vi "rad_Create AppImage Info File.vi"(8 "error in (no error)":errorcluster, 10 "Temp Image Folder":path, 11 "AppImage Properties":T1) -> (0 "error out":errorcluster, 3 "App Image Info file path":path)   [LabVIEW 2020]
uses:
  TypeDefs/rad_Application Image Properties.ctl
  TypeDefs/rad_FPGA Properties.ctl
  TypeDefs/rad_FPGA Flash Properties.ctl
  rad_Globals.vi
  <vilib>/Utility/config.llb/Write Key (String).vi
  <vilib>/Utility/config.llb/NI_LVConfig.lvlib
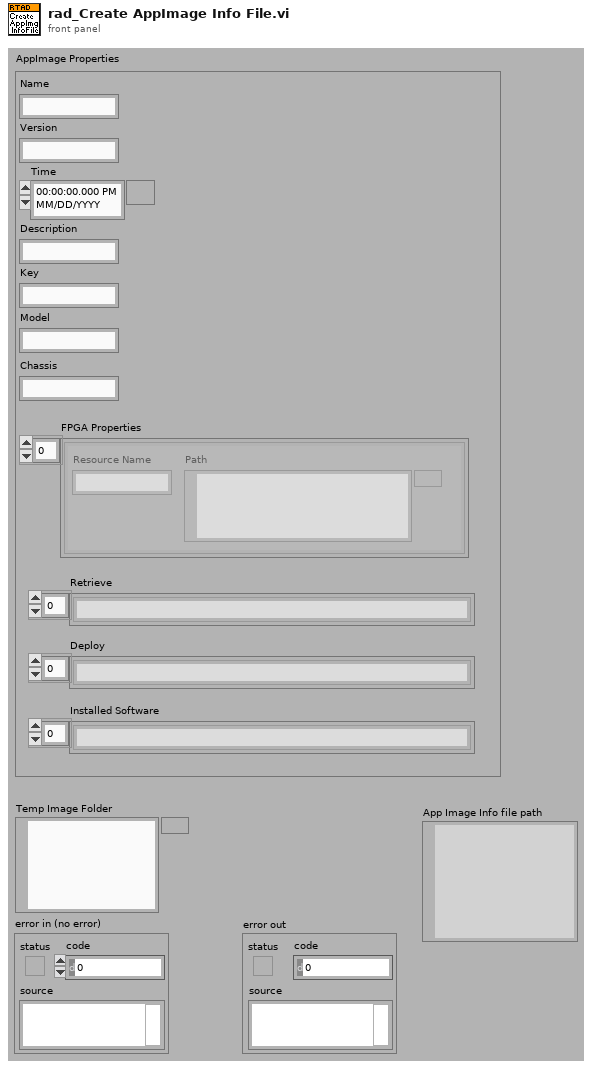
[diagram p1: front panel]
types:
  T1 = typedef "rad_Application Image Properties.ctl" = cluster{"Name":string, "Version":string, "Time":timestamp, "Description":string, "Key":string, "Chassis":string, "FPGA Properties":T2, "Model":string, "Retrieve":string[], "Deploy":string[], "Installed Software":string[]}
  T2 = typedef "rad_FPGA Properties.ctl" = T3[]
  T3 = typedef "rad_FPGA Flash Properties.ctl" = cluster{"Resource Name":string, "Path":path}
  T4 = typedef "NI_LVConfig.lvlib/Config Data RefNum.ctl" = refnum<k1>
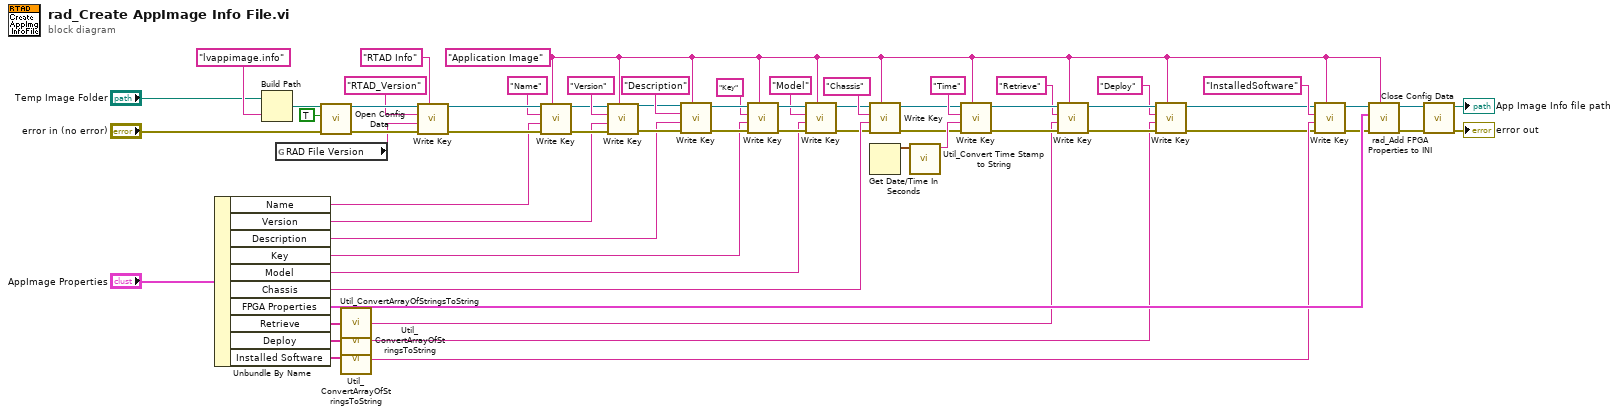
[diagram p0: block diagram]
diagram:
  w6 = "Application Image" ("section")
  n1 = Unbundle By Name("AppImage Properties") -> ("Name"=w41:string, "Version"=w40:string, "Description"=w30:string, "Key"=w29:string, "Model"=w21:string, "Chassis"=w31:string, "FPGA Properties"=w26:T2, "Retrieve"=w13:string[], "Deploy"=w12:string[], "Installed Software"=w8:string[])
  n2 = Build Path(base path="Temp Image Folder", name or relative path="lvappimage.info") -> (appended path=w53:path)
  n3 = global read "rad_Globals.vi" "RAD File Version"() -> (w38:string)
  n4 = call <vilib>:"Open Config Data.vi"("error in (no error)"="error in (no error)", "create file if necessary (T)"=TRUE, "configuration file path"=w53) -> ("error out"=w58:errorcluster, "refnum"=w57:T4)  [unwired: 6 in, 1 out]
  n5 = call "Util_ConvertArrayOfStringsToString.vi"("Array<string>"=w13) -> ("String"=w11:string)
  n6 = call "Util_ConvertArrayOfStringsToString.vi"("Array<string>"=w12) -> ("String"=w10:string)
  n7 = call "Util_ConvertArrayOfStringsToString.vi"("Array<string>"=w8) -> ("String"=w7:string)
  n8 = call-poly <vilib>:"Write Key.vi"("section"="RTAD Info", "error in (no error)"=w58, "value"=w38, "key"="RTAD_Version", "refnum"=w57) -> ("error out"=w59:errorcluster, "refnum out"=w60:T4)  [unwired: 1 in, 4 out]
  n9 = call-poly <vilib>:"Write Key.vi"("section"=w6, "error in (no error)"=w59, "value"=w41, "key"="Name", "refnum"=w60) -> ("error out"=w46:errorcluster, "refnum out"=w47:T4)  [unwired: 1 in, 4 out]
  n10 = call-poly <vilib>:"Write Key.vi"("section"=w6, "error in (no error)"=w46, "value"=w40, "key"="Version", "refnum"=w47) -> ("error out"=w49:errorcluster, "refnum out"=w50:T4)  [unwired: 1 in, 4 out]
  n11 = call-poly <vilib>:"Write Key.vi"("section"=w6, "error in (no error)"=w49, "value"=w30, "key"="Description", "refnum"=w50) -> ("error out"=w36:errorcluster, "refnum out"=w37:T4)  [unwired: 1 in, 4 out]
  n12 = call-poly <vilib>:"Write Key.vi"("section"=w6, "error in (no error)"=w36, "value"=w29, "key"="Key", "refnum"=w37) -> ("error out"=w23:errorcluster, "refnum out"=w25:T4)  [unwired: 1 in, 4 out]
  n13 = call-poly <vilib>:"Write Key.vi"("section"=w6, "error in (no error)"=w23, "value"=w21, "key"="Model", "refnum"=w25) -> ("error out"=w22:errorcluster, "refnum out"=w24:T4)  [unwired: 1 in, 4 out]
  n14 = call-poly <vilib>:"Write Key.vi"("section"=w6, "error in (no error)"=w22, "value"=w31, "key"="Chassis", "refnum"=w24) -> ("error out"=w34:errorcluster, "refnum out"=w33:T4)  [unwired: 1 in, 4 out]
  n15 = Get Date/Time In Seconds() -> (seconds since 1Jan1904=w61:timestamp)
  n16 = call "Util_Convert Time Stamp to String.vi"("Time"=w61) -> ("Time"=w63:string)  [unwired: 10 out]
  n17 = call-poly <vilib>:"Write Key.vi"("section"=w6, "error in (no error)"=w34, "value"=w63, "key"="Time", "refnum"=w33) -> ("error out"=w19:errorcluster, "refnum out"=w17:T4)  [unwired: 1 in, 4 out]
  n18 = call-poly <vilib>:"Write Key.vi"("section"=w6, "error in (no error)"=w19, "value"=w11, "key"="Retrieve", "refnum"=w17) -> ("error out"=w18:errorcluster, "refnum out"=w16:T4)  [unwired: 1 in, 4 out]
  n19 = call-poly <vilib>:"Write Key.vi"("section"=w6, "error in (no error)"=w18, "value"=w10, "key"="Deploy", "refnum"=w16) -> ("error out"=w2:errorcluster, "refnum out"=w5:T4)  [unwired: 1 in, 4 out]
  n20 = call-poly <vilib>:"Write Key.vi"("section"=w6, "error in (no error)"=w2, "value"=w7, "key"="InstalledSoftware", "refnum"=w5) -> ("error out"=w3:errorcluster, "refnum out"=w4:T4)  [unwired: 1 in, 4 out]
  n21 = call "rad_Add FPGA Properties to INI.vi"("section"=w6, "error in (no error)"=w3, "FPGA Properties"=w26, "refnum in"=w4) -> ("error out"=w27:errorcluster, "refnum out"=w28:T4)  [unwired: 6 in]
  n22 = call <vilib>:"Close Config Data.vi"("error in (no error)"=w27, "refnum"=w28) -> ("error out"=→"error out":errorcluster, "file path"=→"App Image Info file path":path)  [unwired: 1 in, 7 out]
